vi "jsonGetErrorPtr.vi"(8 "error in (no error)":errorcluster) -> (0 "error out":errorcluster, 2 "return type":i64)   [LabVIEW 2016, in "JSON Document.lvclass"]
uses:
  API/JSON Document Class/JSON Document.lvclass
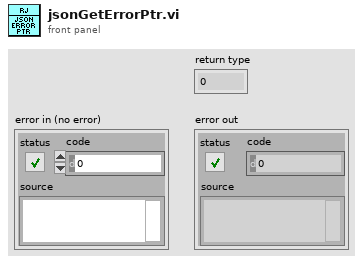
[diagram p1: front panel]
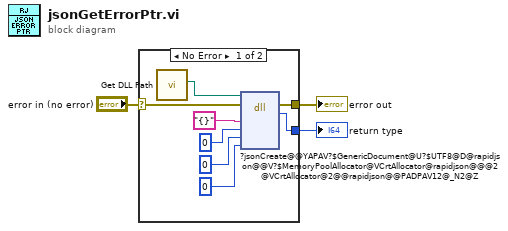
[diagram p0: block diagram]
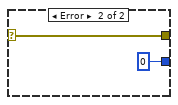
[diagram p2: hidden frame]
diagram:
  n1 = case shown="No Error" "error in (no error)" {
    selector: "error in (no error)" -> [w9 w13]
    tunnel: [w10 i64 0 ("return type")] -> w3
    tunnel: [w8 w13] -> w2
    frame No Error {
      n2 = call "Get DLL Path.vi"() -> ("Path"=w11:path)  [unwired: 11 in]
      n3 = dll-call lib="C:/Users/tblair/Documents/Git Projects/rapidjson-for-LabVIEW/lvrjs/Debug/lvrjs.dll" fn="?jsonCreate@@YAPAV?$GenericDocument@U?$UTF8@D@rapidjson@@V?$MemoryPoolAllocator@VCrtAllocator@rapidjson@@@2@VCrtAllocator@2@@rapidjson@@PADPAV12@_N2@Z"(path in=w11, error in=w9, "json"="{}", "jsonError"=i64 0, "allowComments"=0, "enableExtensions"=0) -> (error out=w8:errorcluster, "return type"=w10:i64)  [unwired: 5 in, 1 out]
    }
    frame Error {
    }
  }
  "return type" <- w3
  "error out" <- w2
